vi "Finish Scan.vi"(7 "Scan finished successfully?":bool, 8 "error in":errorcluster, 11 "Scan Driver.lvclass in":refnum<class "Scan Driver.lvclass">) -> (0 "error out":errorcluster, 3 "Scan Driver.lvclass out":refnum<class "Scan Driver.lvclass">)   [LabVIEW 2009, in "Scan Driver.lvclass"]
doc: "Reset the scan and all Scanners and Readers. Write the data file. Prepare to scan again if more than one scan is requested."
uses:
  Scan Driver.lvclass
  Global/Sound Files.vi
  Scan Driver.lvclass/Scan Driver.ctl
  Scanners/Scanner/Scanner.lvclass
  File IO/File IO.lvclass
  <vilib>/Utility/xml.llb/Write to XML File(string).vi
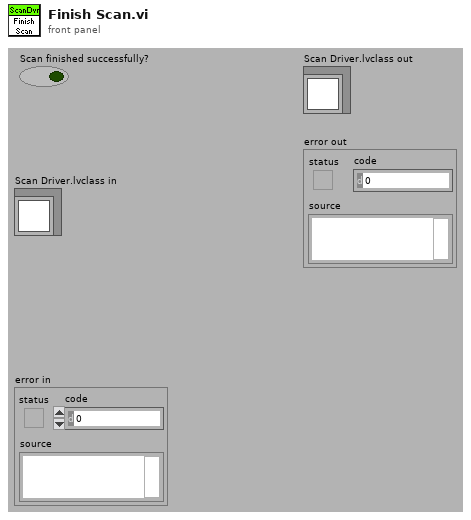
[diagram p1: front panel]
types:
  T1 = typedef "Readable.lvclass/Data Point.ctl" = dbl
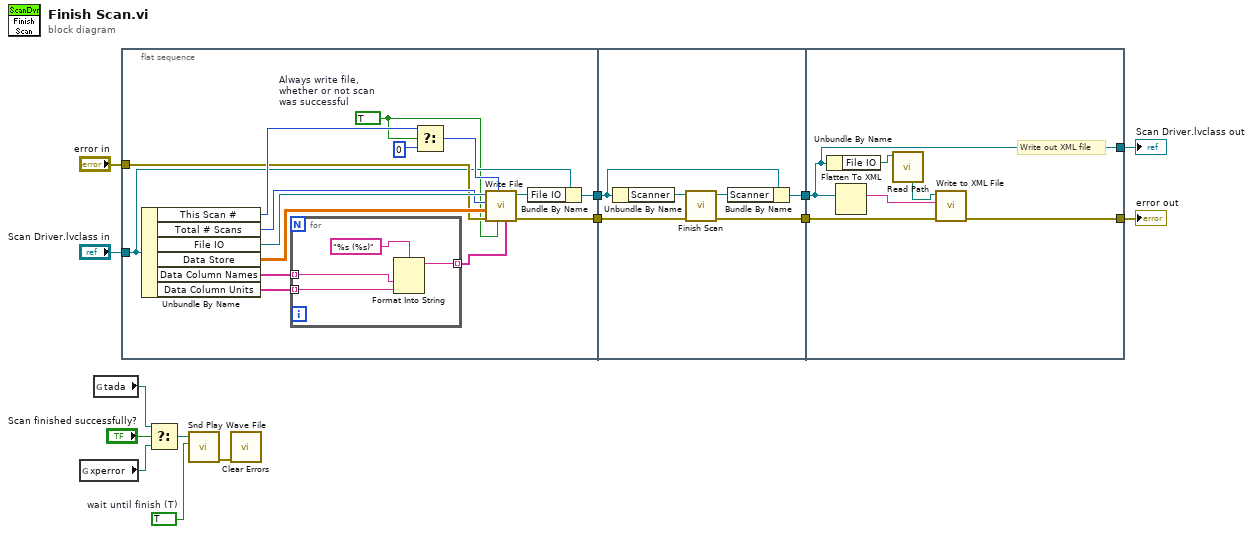
[diagram p0: block diagram]
diagram:
  w5 = TRUE  # wait until finish (T)
  n1 = global read "Sound Files.vi" "xperror"() -> (w2:path)
  n2 = global read "Sound Files.vi" "tada"() -> (w3:path)
  n3 = flat-sequence {
    tunnel: "error in" -> [w22]
    tunnel: "Scan Driver.lvclass in" -> [w21]
    tunnel: [w20] -> w10
    tunnel: [w19] -> w9
    tunnel: w10 -> [w37]
    tunnel: w9 -> [w36]
    tunnel: [w35] -> w8
    tunnel: [w34] -> w7
    tunnel: [w43] -> w14
    tunnel: [w41] -> w12
    tunnel: w8 -> [w41]
    tunnel: w7 -> [w40]
    frame #0 {
      w15 = TRUE  # Always write file, whether or not scan  was successful
      n4 = Unbundle By Name(w21) -> ("This Scan #"=w24:u32, "Total # Scans"=w23:u32, "File IO"=w26:refnum<class "File IO.lvclass">, "Data Store"=w28:T1[][], "Data Column Names"=w17:string[], "Data Column Units"=w18:string[])
      n5 = for {
        tunnel: w18 -> [w32] mode=indexing
        tunnel: w17 -> [w31] mode=indexing
        tunnel: [w30] -> w16 mode=indexing
        n6 = Format Into String(format string="%s (%s)", w31, w32) -> (resulting string=w30:string)  [unwired: 2 in, 1 out]
      }
      n7 = Select(t=w24, s=w15, f=0) -> (s? t:f=w25:u32)
      n8 = call "Write File.vi"("Data Column Headings"=w16, "Write Last Run? (F)"=w15, "Current Scan #"=w25, "error in"=w22, "arraytotaldata"=w28, "#scans"=w23, "File IO in"=w26) -> ("errorOUT"=w19:errorcluster, "File IO out"=w27:refnum<class "File IO.lvclass">)  [unwired: 3 out]
      n9 = Bundle By Name(cluster=w21, "File IO"=w27) -> (w20:refnum<class "Scan Driver.lvclass">)
    }
    frame #1 {
      n10 = Unbundle By Name(w37) -> ("Scanner"=w39:refnum<class "Scanner.lvclass">)
      n11 = call-dynamic "Finish Scan.vi"("error in (no error)"=w36, "Scanner in"=w39) -> ("error out"=w34:errorcluster, "Scanner out"=w38:refnum<class "Scanner.lvclass">)  [unwired: 8 out]
      n12 = Bundle By Name(cluster=w37, "Scanner"=w38) -> (w35:refnum<class "Scan Driver.lvclass">)
    }
    frame #2 {
      # "Write out XML file"
      n13 = Unbundle By Name(w41) -> ("File IO"=w44:refnum<class "File IO.lvclass">)
      n14 = Flatten To XML(anything=w41) -> (xml string=w45:string)
      n15 = call-dynamic "Read Path.vi"("File IO.lvclass in"=w44) -> ("Settings Path"=w42:path)  [unwired: 1 in, 9 out]
      n16 = call-poly <vilib>:"Write to XML File.vi"("error in (no error)"=w40, "XML Input"=w45, "XML File Path"=w42) -> ("error out"=w43:errorcluster)  [unwired: 2 in, 6 out]
    }
  }
  n17 = Select(t=w3, s="Scan finished successfully?", f=w2) -> (s? t:f=w4:path)
  n18 = call <vilib>:"Snd Play Wave File.vi"("wait until finish (T)"=w5, "wave file path"=w4) -> ("error out"=w6:errorcluster)  [unwired: 1 in, 8 out]
  n19 = call <vilib>:"Clear Errors.vi"("error in (no error)"=w6) -> ()  [unwired: 7 out]
  "error out" <- w14
  "Scan Driver.lvclass out" <- w12
